vi "SendCmd_Tool.vi"(5 "path_bat":path=path "C:/Users/user/Desktop/tool/5.bat", 7 "error in (no error) 2":errorcluster) -> (3 "VQT":string, 4 "return code":i32, 6 "Other":string, 8 "release version:":string, 10 "Led Test":string, 13 "standard output":string, 14 "error out 3":errorcluster, 15 "version info":string)   [LabVIEW 2017]
panel:
  out "Reflection":string
  # "[Uniformity]\nInitial brightness : 3.5%\nMean uniformity    : 210.0359\nDeviation          : 79.49728304281851\n\n[Uniformity]\nInitial brightness : 3.5%\nMean uniformity    : 209.5895\nDeviation          : 80.05396673338554\nAdjusted brightness: 4.0%\nMean uniformity    : 213.8874\nDeviation          : 78.03311169779147\nResult             : FAIL"
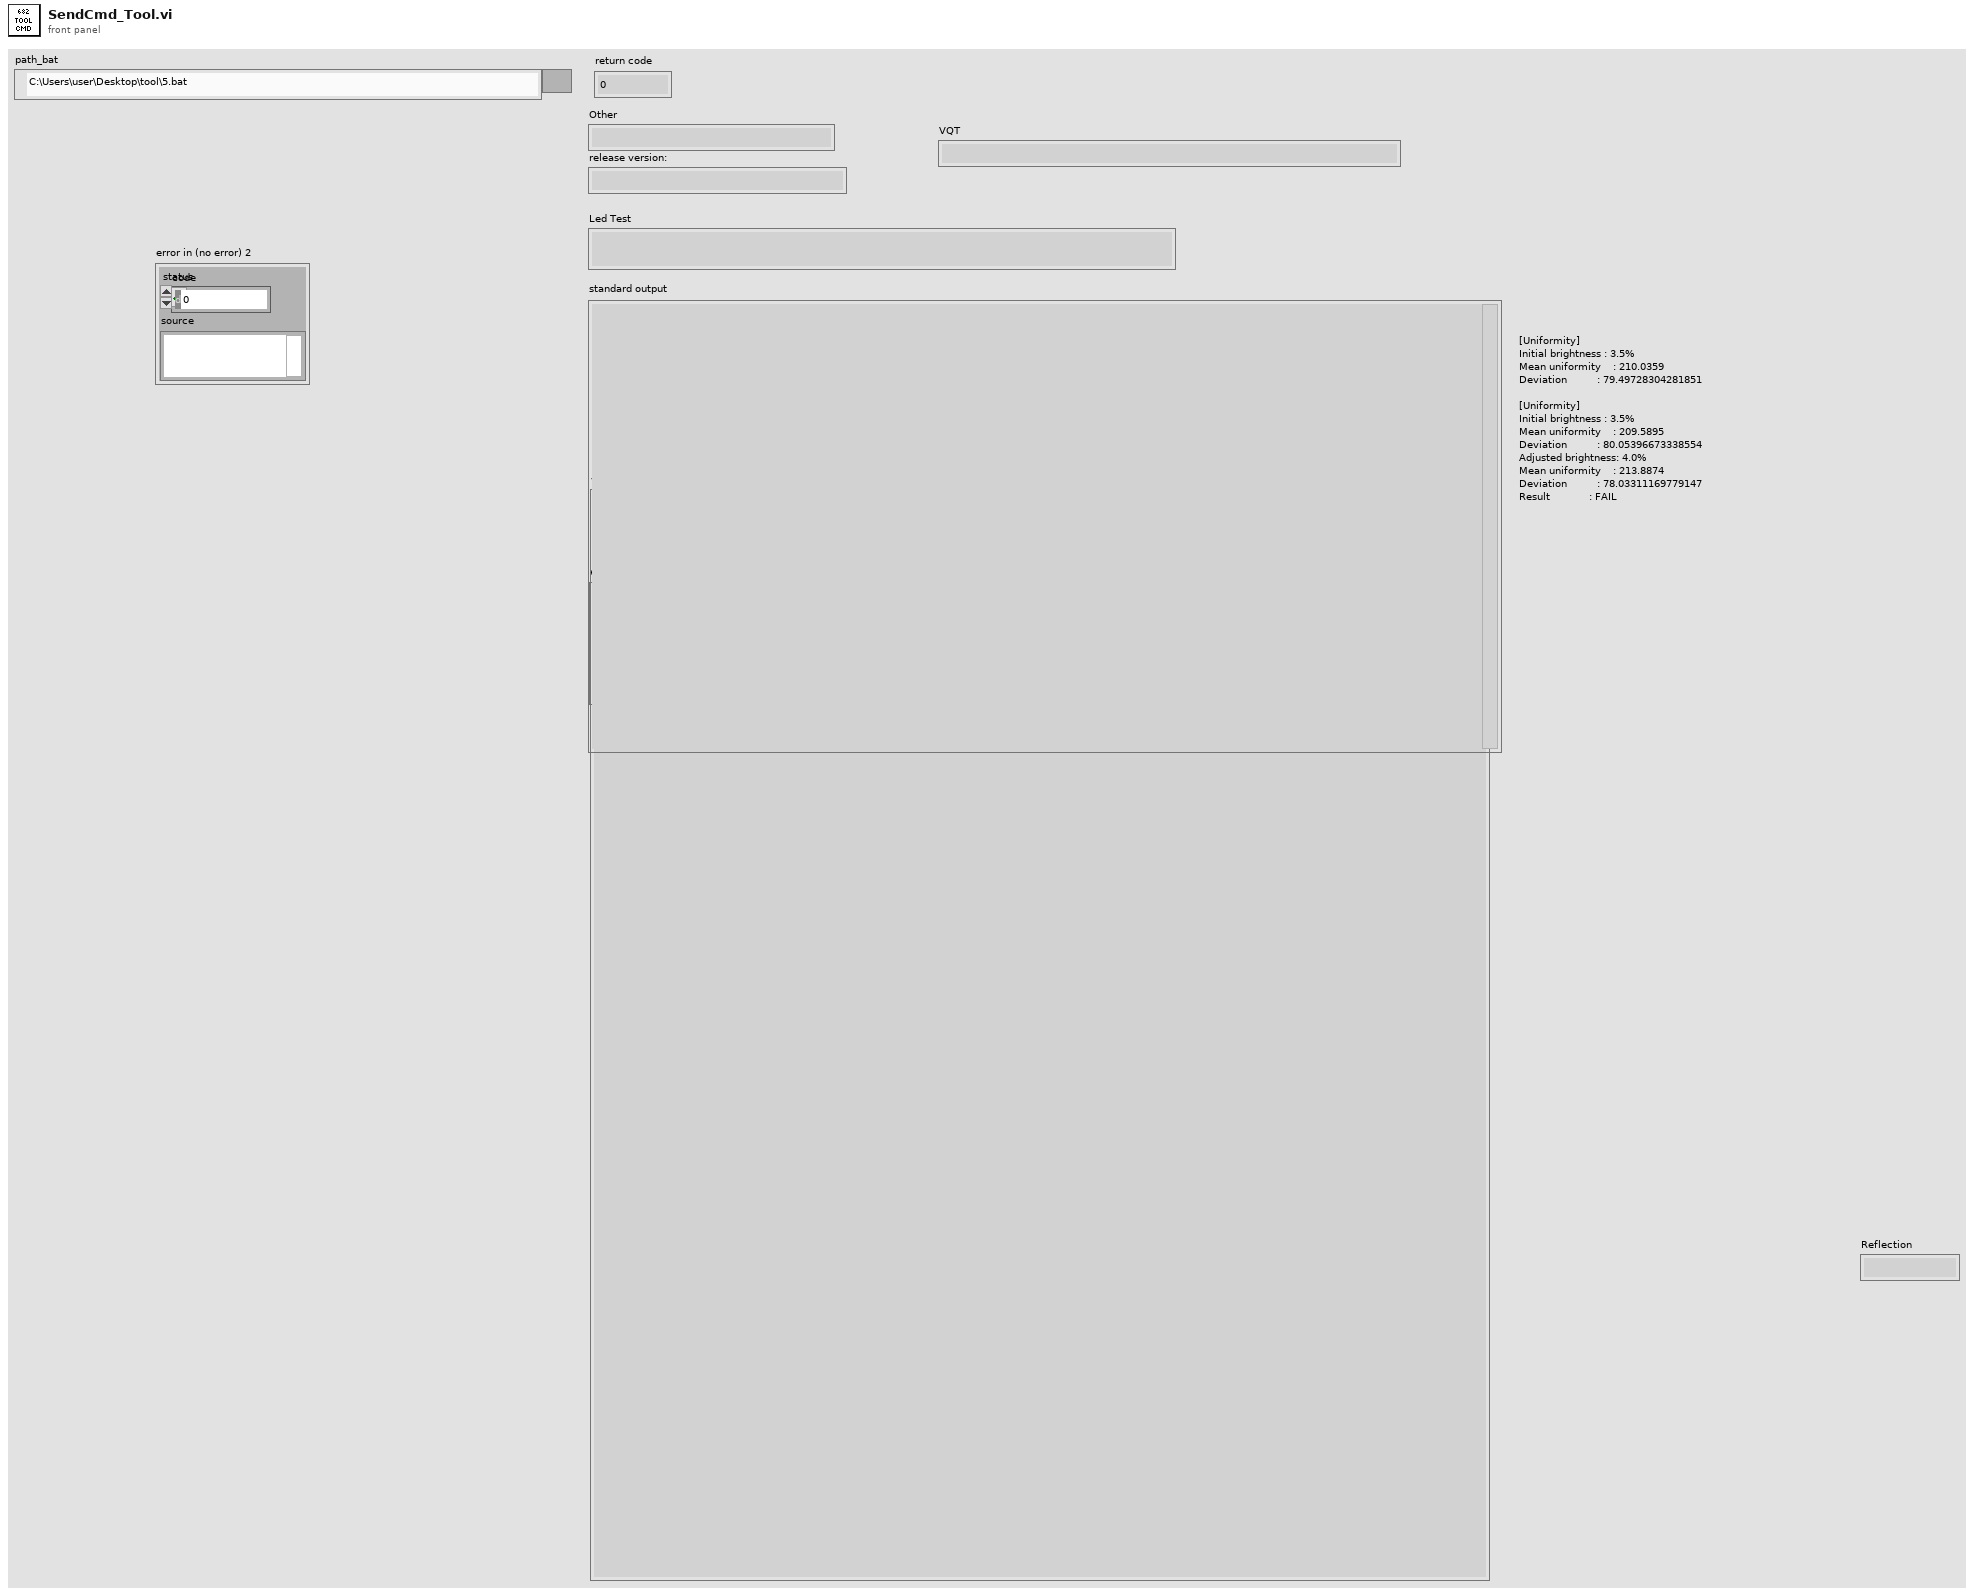
[diagram p1: front panel]
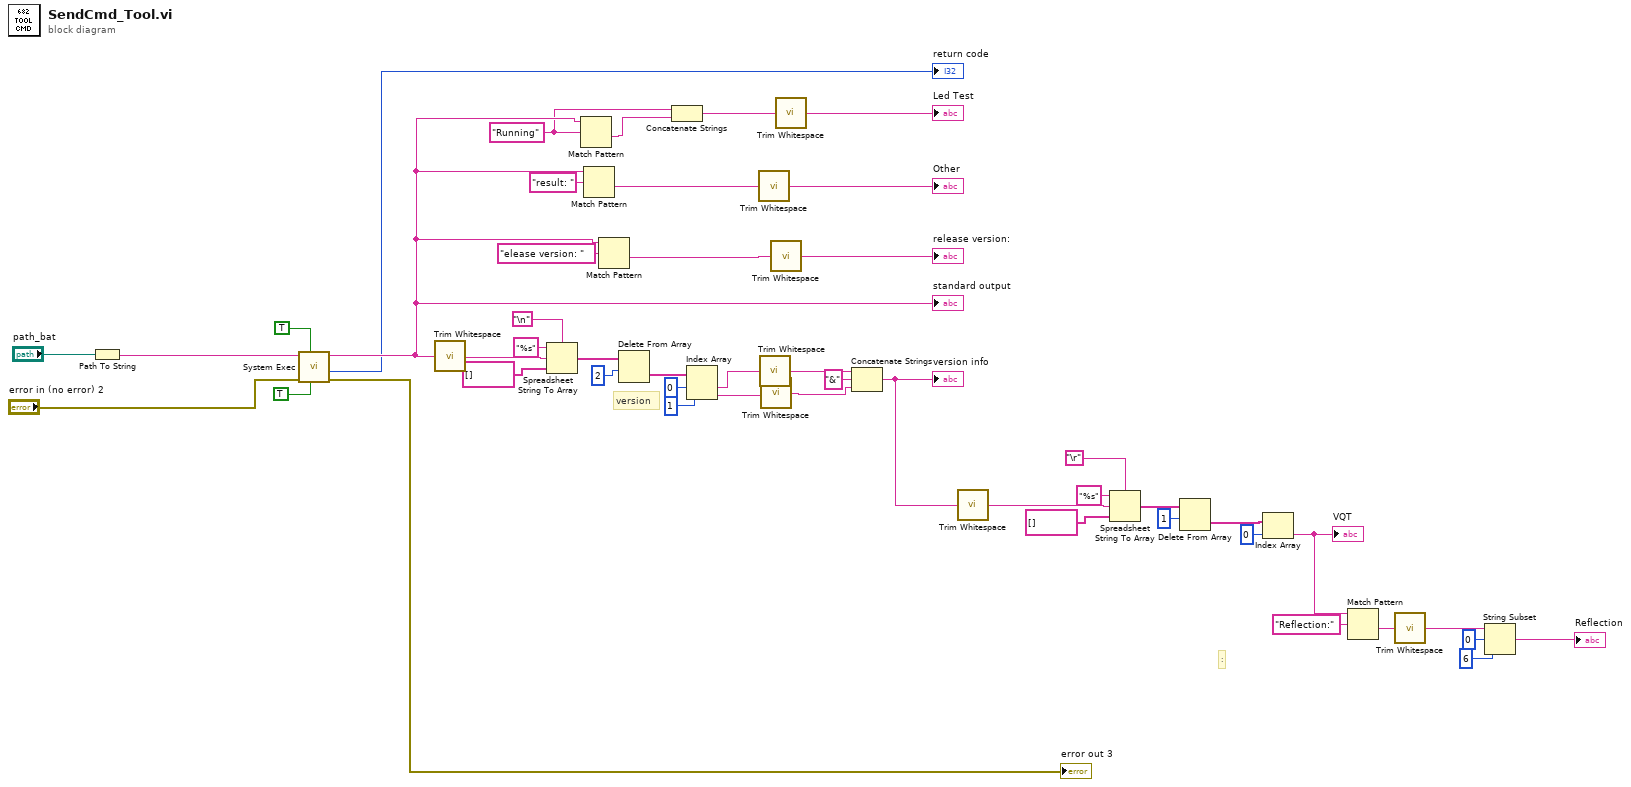
[diagram p0: block diagram]
diagram:
  w24 = "Running" ("regular expression")
  # ":"
  # "version"
  n1 = Path To String(path="path_bat") -> (string=w46:string)
  n2 = call <vilib>:"System Exec.vi"("run minimized? (F)"=TRUE, "wait until completion? (T)"=TRUE, "error in (no error)"="error in (no error) 2", "command line"=w46) -> ("error out"=→"error out 3":errorcluster, "return code"=→"return code":i32, "standard output"=w42:string)  [unwired: 2 in, 3 out]
  "standard output" <- w42
  n3 = call <vilib>:"Trim Whitespace.vi"("string"=w42) -> ("trimmed string"=w37:string)  [unwired: 1 in]
  n4 = Spreadsheet String To Array(delimiter (Tab)="\n", format string="%s", spreadsheet string=w37, array type (2D Dbl)=string[] []) -> (array=w36:string[])
  n5 = Match Pattern(string=w42, regular expression=w24) -> (after substring=w23:string)  [unwired: 1 in, 3 out]
  n6 = Match Pattern(string=w42, regular expression="result: ") -> (after substring=w20:string)  [unwired: 1 in, 3 out]
  n7 = Match Pattern(string=w42, regular expression="elease version: ") -> (after substring=w18:string)  [unwired: 1 in, 3 out]
  n8 = Delete From Array(array=w36, length=2 ("index")) -> (deleted portion=w34:string[])  [unwired: 1 in, 1 out]
  n9 = Concatenate Strings(w24, w23) -> (w22:string)
  n10 = Index Array(array=w34, index #1=0 ("index"), index #2=1 ("index")) -> (element #1=w30:string, element #2=w28:string)
  n11 = call <vilib>:"Trim Whitespace.vi"("string"=w20) -> ("trimmed string"=→"Other":string)  [unwired: 1 in]
  n12 = call <vilib>:"Trim Whitespace.vi"("string"=w30) -> ("trimmed string"=w29:string)  [unwired: 1 in]
  n13 = call <vilib>:"Trim Whitespace.vi"("string"=w28) -> ("trimmed string"=w27:string)  [unwired: 1 in]
  n14 = call <vilib>:"Trim Whitespace.vi"("string"=w18) -> ("trimmed string"=→"release version:":string)  [unwired: 1 in]
  n15 = call <vilib>:"Trim Whitespace.vi"("string"=w22) -> ("trimmed string"=→"Led Test":string)  [unwired: 1 in]
  n16 = Concatenate Strings(w29, "&" ("string"), w27) -> (w8:string)
  "version info" <- w8
  n17 = call <vilib>:"Trim Whitespace.vi"("string"=w8) -> ("trimmed string"=w13:string)  [unwired: 1 in]
  n18 = Spreadsheet String To Array(delimiter (Tab)="\r", format string="%s", spreadsheet string=w13, array type (2D Dbl)=string[] []) -> (array=w12:string[])
  n19 = Delete From Array(array=w12, length=1) -> (deleted portion=w10:string[])  [unwired: 1 in, 1 out]
  n20 = Index Array(array=w10, index=0) -> (element=w1:string)
  "VQT" <- w1
  n21 = Match Pattern(string=w1, regular expression="Reflection:") -> (after substring=w6:string)  [unwired: 1 in, 3 out]
  n22 = call <vilib>:"Trim Whitespace.vi"("string"=w6) -> ("trimmed string"=w5:string)  [unwired: 1 in]
  n23 = String Subset(string=w5, offset (0)=0, length (rest)=6 ("length (rest)")) -> (substring=→"Reflection":string)
